vi "DT3120_AquireFrame.vi"(8 "error in (no error)":errorcluster, 9 "Image":T1, 10 "Frame Size":T2, 11 "DevId":i32) -> (0 "error out":errorcluster, 1 "Image Out":T1, 2 "Frame":u8[][](array[numeric]), 3 "DevId (dup)":i32)   [LabVIEW 2013]
uses:
  <vilib>/vision/Image Controls.llb/IMAQ Image.ctl
  olfg32.dll
panel:
  out "BufSize":u32
  out "FrameId":u32
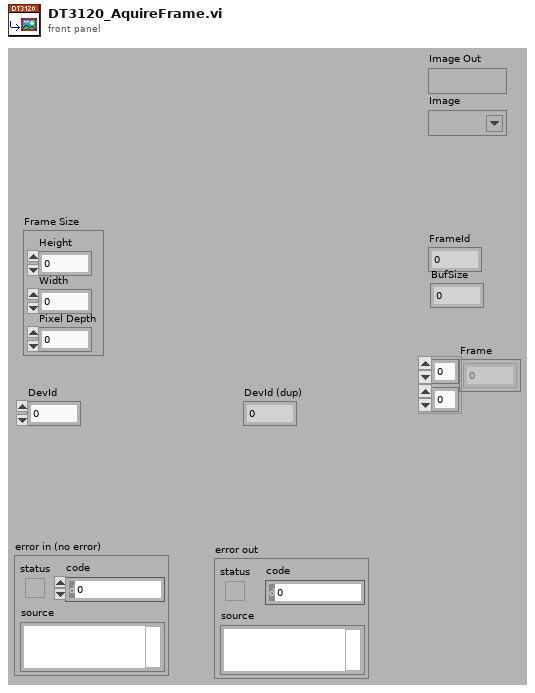
[diagram p1: front panel]
types:
  T1 = typedef "IMAQ Image.ctl" = refnum<image>
  T2 = cluster{"Height":u32, "Width":u32, "Pixel Depth":u32}
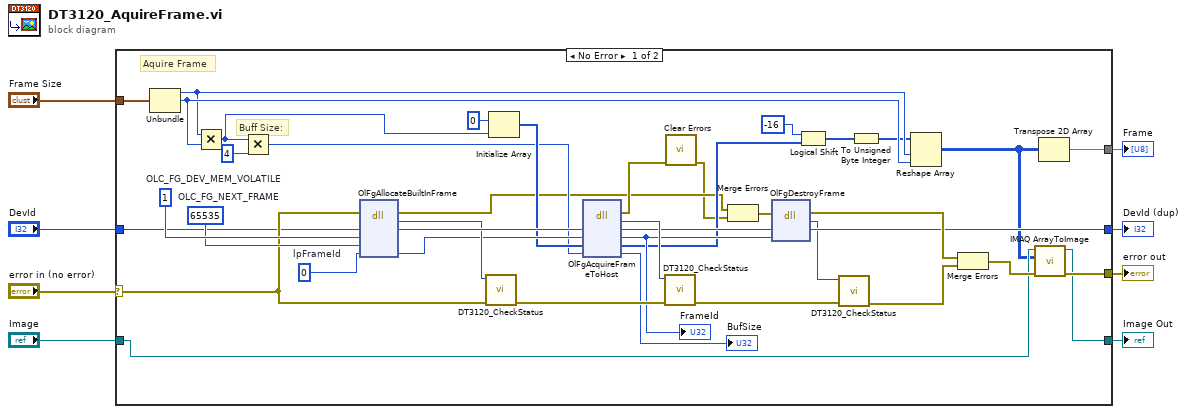
[diagram p0: block diagram]
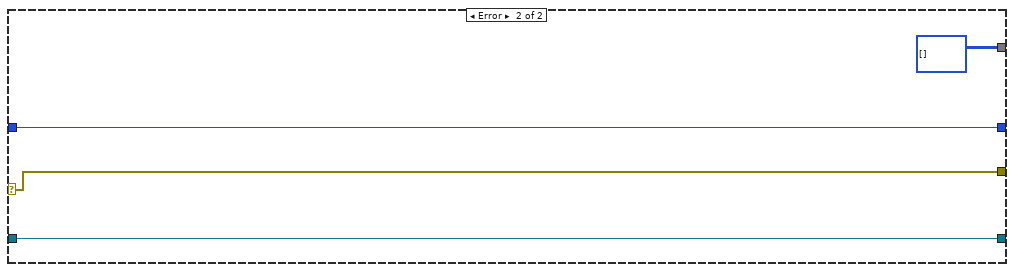
[diagram p2: hidden frame]
diagram:
  n1 = case shown="No Error" "error in (no error)" {
    selector: "error in (no error)" -> [w40 w52]
    tunnel: "DevId" -> [w39 w51]
    tunnel: [w19 w52] -> w7
    tunnel: [w27 w51] -> w6
    tunnel: "Frame Size" -> [w46 _]
    tunnel: [w13 u8[][] [] ("lpBuffer")] -> w3
    tunnel: [w18 w49] -> w2
    tunnel: "Image" -> [w17 w49]
    frame No Error {
      w41 = u32 0  # lpFrameId
      w42 = u16 65535  # OLC_FG_NEXT_FRAME
      w43 = 1  # OLC_FG_DEV_MEM_VOLATILE
      # "Buff Size:"
      # "Aquire Frame"
      n2 = Unbundle(w46) -> ("Height"=w33:u32, "Width"=w34:u32)  [unwired: 1 out]
      n3 = Multiply(x=w33, y=w34) -> (x*y=w30:u32)
      n4 = Multiply(x=w30, y=u32 4) -> (x*y=w31:u32)
      n5 = dll-call lib="C:/Users/dhaehnel/Documents/Workspace/Labview_Workspace/labviewlib/MT Scan/SubVIs/olfg32.dll" fn="OlFgAllocateBuiltInFrame"(error in=w40, "DevId"=w39, "MemType"=w43, "BufNum"=w42, "lpFrameId"=w41) -> (error out=w11:errorcluster, "Status"=w37:u32, "DevId"=w38:i32, "lpFrameId"=w36:u32)  [unwired: 4 in, 1 out]
      n6 = call "DT3120_CheckStatus.vi"("error in"=w40, "Status"=w37) -> ("error out"=w48:errorcluster)  [unwired: 9 out]
      n7 = Initialize Array(u32 0 ("element"), w30) -> (w35:u32[])
      n8 = dll-call lib="C:/Users/dhaehnel/Documents/Workspace/Labview_Workspace/labviewlib/MT Scan/SubVIs/olfg32.dll" fn="OlFgAcquireFrameToHost"("DevId"=w38, "FrameId"=w36, "lpBuffer"=w35, "BufSize"=w31) -> (error out=w12:errorcluster, "Status"=w47:u32, "DevId"=w28:i32, "FrameId"=w26:u32, "lpBuffer"=w22:u32[], "BufSize"=→"BufSize":u32)  [unwired: 3 in, 1 out]
      "FrameId" <- w26
      n9 = call "DT3120_CheckStatus.vi"("error in"=w48, "Status"=w47) -> ("error out"=w24:errorcluster)  [unwired: 9 out]
      n10 = call <vilib>:"Clear Errors.vi"("error in (no error)"=w12) -> ("error out"=w9:errorcluster)  [unwired: 6 in]
      n11 = Merge Errors(w11, w9) -> (w10:errorcluster)
      n12 = dll-call lib="C:/Users/dhaehnel/Documents/Workspace/Labview_Workspace/labviewlib/MT Scan/SubVIs/olfg32.dll" fn="OlFgDestroyFrame"(error in=w10, "DevId"=w28, "FrameId"=w26) -> (error out=w29:errorcluster, "Status"=w25:u32, "DevId"=w27:i32)  [unwired: 3 in, 1 out]
      n13 = Logical Shift(y=i8 -16, x=w22) -> (x << y=w16:u32[])
      n14 = call "DT3120_CheckStatus.vi"("error in"=w24, "Status"=w25) -> ("error out"=w23:errorcluster)  [unwired: 9 out]
      n15 = To Unsigned Byte Integer(number=w16) -> (unsigned 8bit integer=w15:u8[])
      n16 = Reshape Array(w15, w33, w34) -> (w14:u8[][])
      n17 = Merge Errors(w29, w23) -> (w20:errorcluster)
      n18 = call "IMAQ ArrayToImage"("error in (no error)"=w20, "Image Pixels (U8)"=w14, "Image"=w17) -> ("error out"=w19:errorcluster, "Image Out"=w18:T1)  [unwired: 7 in]
      n19 = Transpose 2D Array(2D array=w14) -> (transposed array=w13:u8[][])
    }
    frame Error {
    }
  }
  "error out" <- w7
  "DevId (dup)" <- w6
  "Frame" <- w3
  "Image Out" <- w2
